vi "Realsense Cam Capture Stop.vi"(8 "error in (no error)":errorcluster, 11 "Realsense Cam in":refnum<class "Realsense Cam.lvclass">) -> (0 "error out":errorcluster, 2 "error":u64, 3 "Realsense Cam out":refnum<class "Realsense Cam.lvclass">)   [LabVIEW 2018, in "Realsense Cam.lvclass"]
uses:
  Realsense Cam.lvclass
  Realsense Cam.lvclass/Realsense Cam.ctl
  realsense_wrapper_api/libRealSense3.lvlib
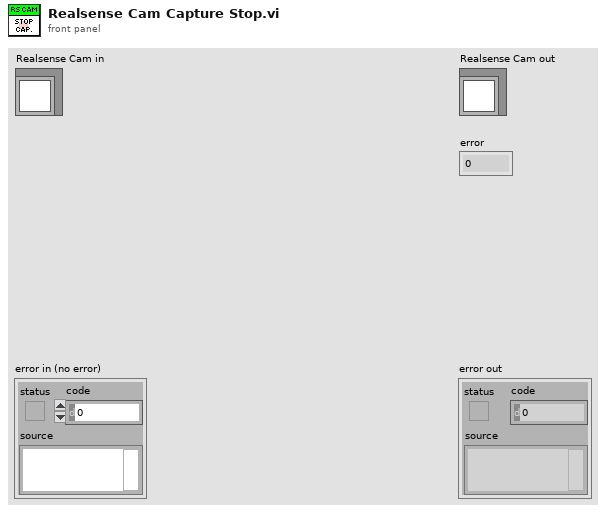
[diagram p1: front panel]
types:
  T1 = cluster{"decimation filter queue":u64, "spatial filter queue":u64, "temporal filter queue":u64, "disparity_transforg_2_queue":u64, "disparity_transforg_1_queue":u64}
  T2 = cluster{"decimation filter block":u64, "spatial filter block":u64, "temporal filter block":u64, "disparity_transforg_2_block":u64, "disparity_transforg_1_block":u64}
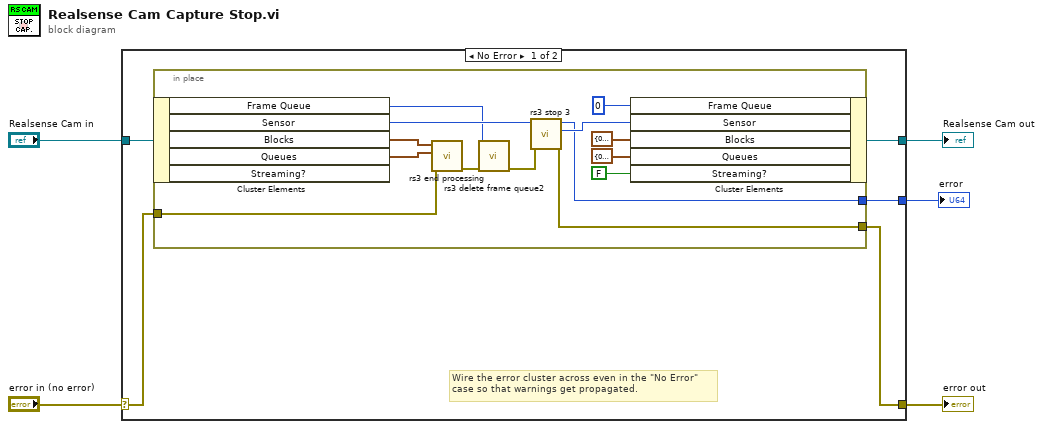
[diagram p0: block diagram]
diagram:
  n1 = case shown="No Error" "error in (no error)" {
    selector: "error in (no error)" -> [w8 w26]
    tunnel: [w7 w26] -> w4
    tunnel: [w9 w25] -> w2
    tunnel: "Realsense Cam in" -> [w10 w25]
    tunnel: [w6 _] -> w1
    frame No Error {
      # "Wire the error cluster across even in the \"No Error\"\ncase so that warnings get propagated."
      n2 = in-place {
        in-place-border: w8 -> [w18]
        in-place-border: [w21] -> w7
        in-place-border: [w22] -> w6
        n3 = in-place-cluster #1(w10) -> ("Frame Queue"=w16:u64, "Sensor"=w24:u64, "Blocks"=w20:T2, "Queues"=w19:T1)  [unwired: 1 out]
        n4 = call "rs3 end processing.vi"("error in (no error)"=w18, "Processing Queues"=w19, "Processing Blocks"=w20) -> ("error out"=w17:errorcluster)  [unwired: 8 in]
        n5 = call "rs3 delete frame queue2.vi"("error in (no error)"=w17, "queue"=w16) -> ("error out"=w15:errorcluster)  [unwired: 9 in]
        n6 = call "rs3 stop 3.vi"("error in (no error)"=w15, "sensor"=w24) -> ("error out"=w21:errorcluster, "sensor out"=w23:u64, "error"=w22:u64)  [unwired: 7 in]
        n7 = in-place-cluster #1("Frame Queue"=u64 0 ("Device Status.Frame Queue"), "Sensor"=w23, "Blocks"=T2 {"decimation filter block"=0, "spatial filter block"=0, "temporal filter block"=0, "disparity_transforg_2_block"=0, "disparity_transforg_1_block"=0} ("Device Status.Settings.Advanced.Post Processing.Processing Blocks"), "Queues"=T1 {"decimation filter queue"=0, "spatial filter queue"=0, "temporal filter queue"=0, "disparity_transforg_2_queue"=0, "disparity_transforg_1_queue"=0} ("Device Status.Settings.Advanced.Post Processing.Processing Queues"), "Streaming?"=FALSE ("Stream Data.Started?")) -> (w9:refnum<class "Realsense Cam.lvclass">)
      }
    }
    frame Error {
    }
  }
  "error out" <- w4
  "Realsense Cam out" <- w2
  "error" <- w1
